vi "test.vi"() -> ()   [LabVIEW 2024]
uses:
  <userlib>/libsocketcan_fd/libsocketcan_fd.lvlib
panel:
  out "data string":string
  in  "stop":bool
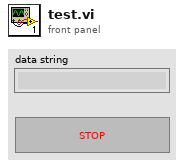
[diagram p1: front panel]
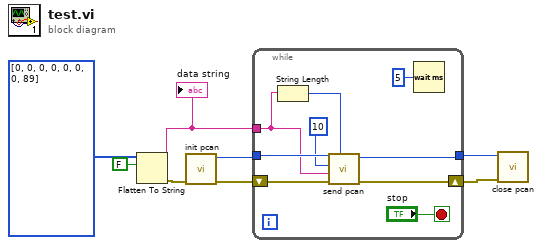
[diagram p0: block diagram]
diagram:
  n1 = Flatten To String(anything=u8[] [0, 0, 0, 0, 0, 0, 0, 89], prepend array or string size? (T)=FALSE) -> (data string=w5:string, error out=w1:errorcluster)  [unwired: 2 in, 1 out]
  "data string" <- w5
  n2 = call <userlib>:"init pcan.vi"("error in (no error)"=w1) -> ("error out"=w7:errorcluster, "function return"=w8:i32)  [unwired: 9 in]
  n3 = while {
    tunnel: w5 -> [w11]
    shift-right: [w15] -> w4
    shift-left: w7 -> [w16]
    tunnel: w8 -> [w17]
    tunnel: [w14] -> w3
    stop <- "stop" stop-if-true
    n4 = String Length(string=w11) -> (length=w9:i32)
    n5 = call <userlib>:"send pcan.vi"("len"=w9, "error in (no error)"=w16, "data"=w11, "can_id"=10, "sock"=w17) -> ("error out"=w15:errorcluster, "function return"=w14:i32)  [unwired: 4 in, 1 out]
    n6 = Wait (ms)(milliseconds to wait=u32 5) -> ()  [unwired: 1 out]
  }
  n7 = call <userlib>:"close pcan.vi"("error in (no error)"=w4, "sock"=w3) -> ()  [unwired: 9 in, 1 out]
